vi "Sound Relative Path.vi"(11 "Sound":string) -> (3 "Relative Path":path)   [LabVIEW 2017]
panel:
  in  "stop":bool
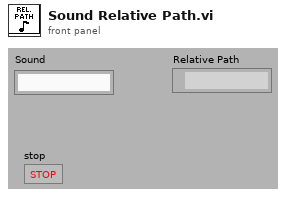
[diagram p1: front panel]
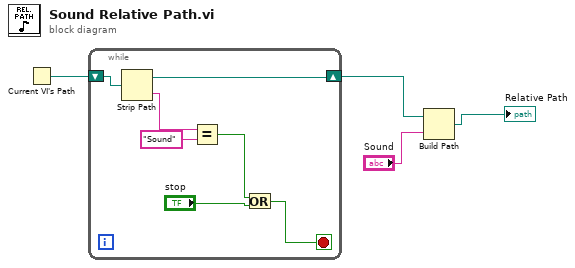
[diagram p0: block diagram]
diagram:
  n1 = Current VI's Path() -> (path=w4:path)
  n2 = while {
    shift-right: [w10] -> w3
    shift-left: w4 -> [w11]
    stop <- w6 stop-if-true
    n3 = Strip Path(path=w11) -> (stripped path=w10:path, name=w5:string)
    n4 = Equal?(x=w5, y="Sound") -> (x = y?=w8:bool)
    n5 = Or(x=w8, y="stop") -> (x .or. y?=w6:bool)
  }
  n6 = Build Path(base path=w3, name or relative path="Sound") -> (appended path=→"Relative Path":path)
